vi "encodeTimeout.vi"(1 "timeout_mclks":u16) -> (0 "reg_val":u16)   [LabVIEW 2018]
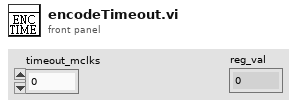
[diagram p1: front panel]
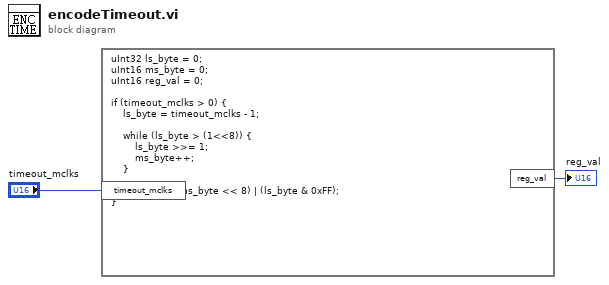
[diagram p0: block diagram]
diagram:
  n1 = formula code="uInt32 ls_byte = 0;\nuInt16 ms_byte = 0;\nuInt16 reg_val = 0;\n\nif (timeout_mclks > 0) {\n    ls_byte = timeout_mclks - 1;\n\n    while (ls_byte > (1<<8)) {\n        ls_byte >>= 1;\n        ms_byte++;\n    }\n\n    reg_val =  (ms_byte << 8) | (ls_byte & 0xFF);\n}"("timeout_mclks"="timeout_mclks") -> ("reg_val"=→"reg_val":u16)
